vi "Read Measurement (Trend Plot Mode).vi"(8 "error in (no error)":errorcluster, 10 "Measurement Type (11: Measurement Reading 1)":i32(ring)=11 items=["Measurement Reading 1"=11, "Measurement Reading 2"=21, "Measurement Reading 3"=31, "Measurement Reading 4"=41], 11 "VISA resource name":refnum<visa-resource-name>) -> (0 "error out":errorcluster, 2 "Measurement Value":dbl format="%#.3e", 3 "VISA resource name out":refnum<visa-resource-name>)   [LabVIEW 2014, in "Fluke 190 Series II.lvlib"]
doc: "Queries the measurement result from the Scopemeter in trend plot mode."
uses:
  Fluke 190 Series II.lvlib
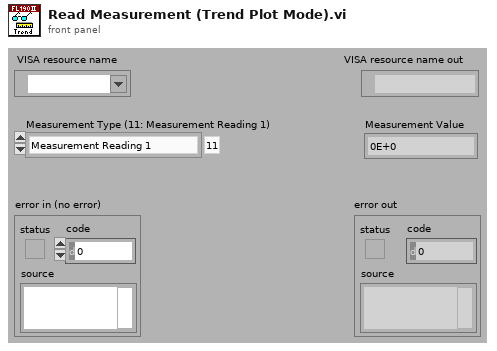
[diagram p1: front panel]
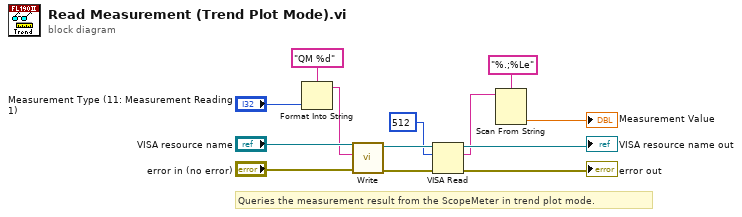
[diagram p0: block diagram]
diagram:
  # "Queries the measurement result from the ScopeMeter in trend plot mode."
  n1 = Format Into String(format string="QM %d", "Measurement Type (11: Measurement Reading 1)") -> (resulting string=w9:string)  [unwired: 2 in, 1 out]
  n2 = call "Write.vi"("error in (no error)"="error in (no error)", "Write Buffer"=w9, "VISA resource name"="VISA resource name") -> ("error out"=w7:errorcluster, "VISA resource name out"=w8:refnum<visa-resource-name>)  [unwired: 7 out]
  n3 = VISA Read(VISA resource name=w8, byte count=u32 512, error in (no error)=w7) -> (VISA resource name out=→"VISA resource name out":refnum<visa-resource-name>, read buffer=w3:string, error out=→"error out":errorcluster)  [unwired: 1 out]
  n4 = Scan From String(format string="%.;%Le", input string=w3) -> (output 1=→"Measurement Value":dbl)  [unwired: 2 in, 4 out]
